vi "SortAssets.vi"(11 "AssetNodes in":T1[](array[typedef])) -> (3 "AssetNodes out":T1[](array[typedef]))   [LabVIEW 2016]
doc: "Queries for all equipment asset nodes, which means they have operating states."
uses:
  <vilib>/addons/InsightCM/MessageBus/Base/controls/AssetState.ctl
  <vilib>/addons/InsightCM/MessageBus/Base/controls/KeyValuePair.ctl
  <vilib>/addons/InsightCM/MessageBus/Base/controls/Metric.ctl
  <vilib>/addons/InsightCM/MessageBus/Base/controls/AssetNodeReference.ctl
  <vilib>/addons/InsightCM/MessageBus/Base/controls/AssetNodeView.ctl
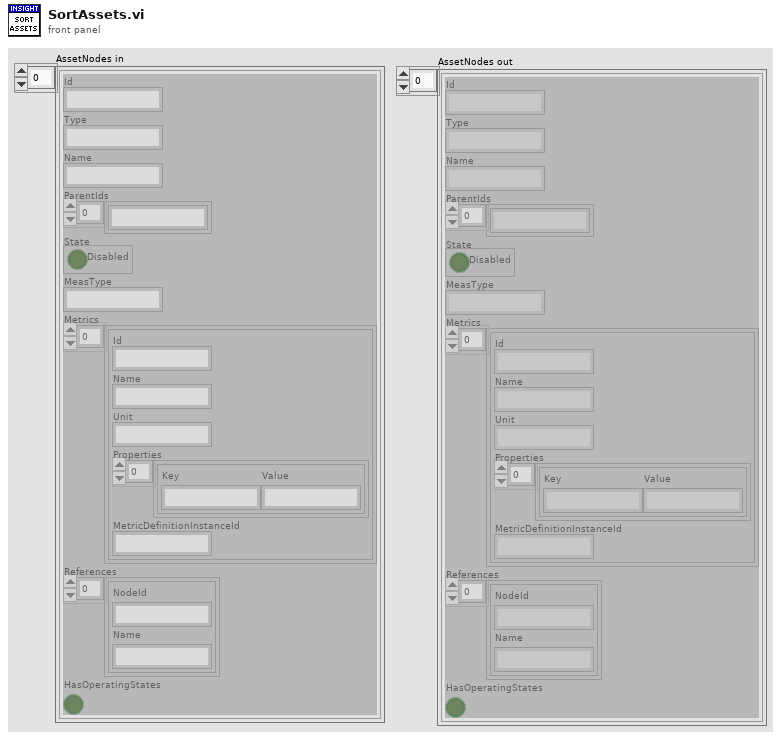
[diagram p1: front panel]
types:
  T1 = typedef "AssetNodeView.ctl" = cluster{"Id":string, "Type":string, "Name":string, "ParentIds":string[], "State":T2, "MeasType":string, "Metrics":T3[], "References":T5[], "HasOperatingStates":bool}
  T2 = typedef "AssetState.ctl" = cluster{"Disabled":bool}
  T3 = typedef "Metric.ctl" = cluster{"Id":string, "Name":string, "Unit":string, "Properties":T4[], "MetricDefinitionInstanceId":string}
  T4 = typedef "KeyValuePair.ctl" = cluster{"Key":string, "Value":string}
  T5 = typedef "AssetNodeReference.ctl" = cluster{"NodeId":string, "Name":string}
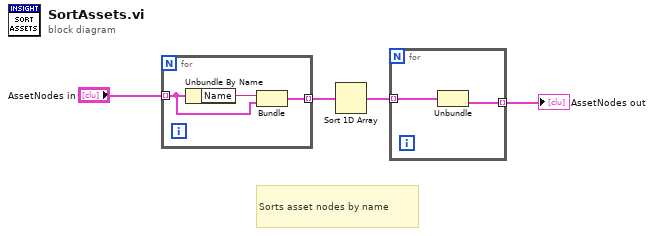
[diagram p0: block diagram]
diagram:
  # "Sorts asset nodes by name"
  n1 = for {
    tunnel: "AssetNodes in" -> [w6] mode=indexing
    tunnel: [w5] -> w3 mode=indexing
    n2 = Unbundle By Name(w6) -> ("Name"=w7:string)
    n3 = Bundle("Name"=w7, "AssetNodeView"=w6) -> (w5:cluster{"Name":string, "AssetNodeView":T1})  [unwired: 1 in]
  }
  n4 = Sort 1D Array(array=w3) -> (sorted array=w2:cluster{"Name":string, "AssetNodeView":T1}[])
  n5 = for {
    tunnel: w2 -> [w9] mode=indexing
    tunnel: [w8] -> w1 mode=indexing
    n6 = Unbundle(w9) -> ("AssetNodeView"=w8:T1)  [unwired: 1 out]
  }
  "AssetNodes out" <- w1
